vi "TTA_MATLAB_RxACPRTest.vi"(1 "Instrument Cluster In":T2, 11 "error in":errorcluster) -> (4 "ACPR\nResults":T1, 12 "Instrument Cluster Out":T2, 15 "error out":errorcluster)   [LabVIEW 2016]
uses:
  TTA_Globals/TTA_Global_Complete_Settings.vi
  TTA_Controls/TTA_Control_Complete_Settings_Cluster.ctl
  TTA_Controls/TTA_Control_Instrument_Cluster.ctl
panel:
  out "Test Status":string
  in  "Complete Settings Cluster":T3
  out "RFICs":i32[](array[numeric])
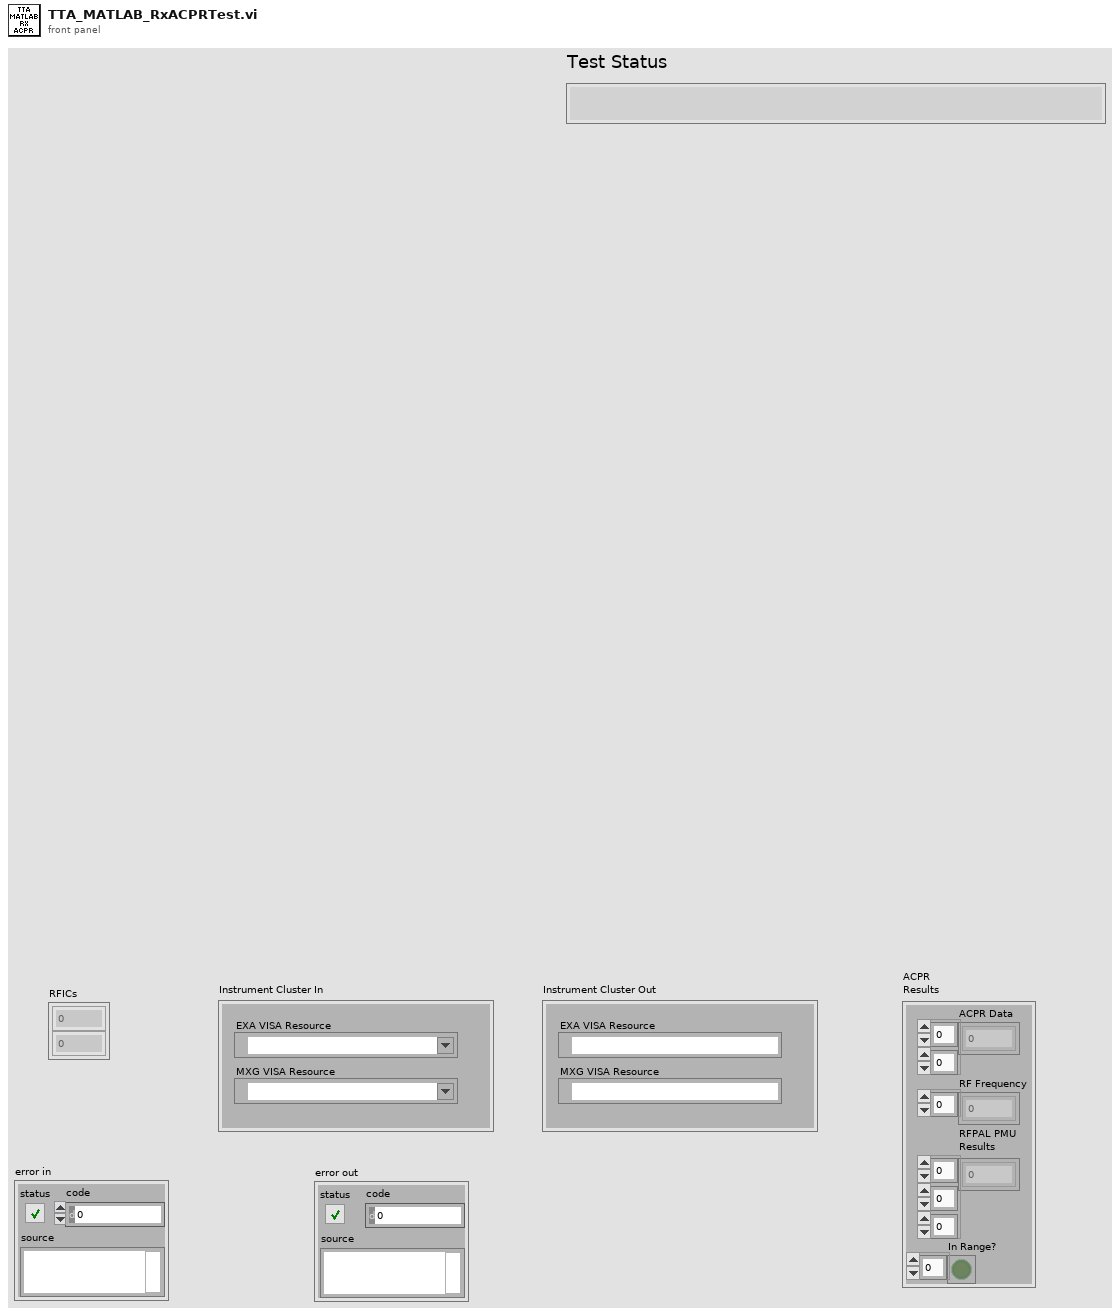
[diagram p1: front panel]
types:
  T1 = cluster{"ACPR Data":dbl[][], "RF Frequency":dbl[], "RFPAL PMU\nResults":dbl[][][], "In Range?":bool[]}
  T2 = typedef "TTA_Control_Instrument_Cluster.ctl" = cluster{"EXA VISA Resource":refnum<visa-resource-name>, "MXG VISA Resource":refnum<visa-resource-name>}
  T3 = typedef "TTA_Control_Complete_Settings_Cluster.ctl" = cluster{"Brief Cluster":cluster{"STM Firmware File":string, "STM Firmware Address":string, "Required SW Version":string, "Template Used":string}, "Instrument Setting Cluster":cluster{"BDSFreq":dbl, "BDS Amp":dbl, "TxRFCal_Freq":dbl, "TxRFCal_Amp":dbl, "RxRFCal_Freq":dbl, "RxRFCal_Freq":dbl, "TxIF_Freq":dbl, "TxIF_Amp":dbl, "Tx_Output_Power_Signal_Freq":dbl, "Tx_ACPR_Signal_Freq":dbl, "Rx_RF_Freq":dbl, "Rx_RF_Amp":dbl, "Rx_Output_Power_Signal_Freq":dbl, "Rx_Output_Power_Sense_Freq":dbl}, "PAL Calibration\nInputs Cluster":cluster{"Amplitude Range\nMax(dBm)":dbl, "Amplitude Range\nMin(dBm)":dbl, "Amplitude Least\nCriteria (dBm)":dbl, "Frequency 1":dbl, "Frequency 2":dbl, "Frequency 3":dbl, "CAL Amplitude\nDecrement (dB)":dbl, "CAL Amplitude\nIncrement(dB)":dbl, "DownloadFile":string}, "TxOffset Cal Cluster":cluster{"Tx1 Offset (dB)":dbl, "Tx2 Offset (dB)":dbl, "Tx3 Offset (dB)":dbl, "Tx4 Offset (dB)":dbl, "Total RF Tx Loss (dB)":dbl}, "RxOffset Cal Cluster":cluster{"Rx1 Offset (dB)":dbl, "Rx2 Offset (dB)":dbl, "Rx3 Offset (dB)":dbl, "Rx4 Offset (dB)":dbl, "Total RF Rx Loss (dB)":dbl}, "TX Output Power Settings Cluster":cluster{"Frequency Sweep (MHz)":dbl[], "Sig Gen \nPower (dBm)":dbl, "Span (kHz)":dbl, "RBW (Hz)":dbl, "Ref Level (dBm)":dbl, "Low Power \nLimit":dbl, "High Power \nLimit":dbl, "DigAtt Max":dbl, "DigAtt Min":dbl}, "Tx ACPR Settings Cluster":cluster{"ACPR Filename":string, "Sampling Rate":dbl, "Power (dBm)":dbl, "IF Frequency Sweep (MHz)":dbl[], "State Name":string, "Mechanical\nAttenuation":dbl, "RefLevel Offset":dbl, "Amplitude Range\nMax (dBm)":dbl, "Amplitude Range\nMin (dBm)":dbl, "Cal Amp \nIncrement (dB)":dbl, "Cal Amp\nDecrement (dB)":dbl}, "Power Cal Cluster":cluster{"Power List (dBm)":dbl[], "Frequency (MHz)":dbl[], "Cal Decrement (dB)":dbl, "Cal Increment (dB)":dbl}, "Rx Received Power Settings Cluster":cluster{"Frequency Sweep (MHz)":dbl[], "Power (dBm)":dbl, "Span (kHz)":dbl, "RBW (Hz)":dbl, "Ref Level":dbl, "Low Power \nLimit (dBm)":dbl, "High Power\nLimit (dBm)":dbl}, "Tx Output Power Criteria Cluster":cluster{"CH1-TX1 \nMin":dbl, "CH1-TX1\nMax":dbl, "CH1-TXx3\nMin ":dbl, "CH1-TXx3\nMax":dbl, "CH2-TX1\nMin":dbl, "CH2-TX1\nMax":dbl, "CH2-TXx3\nMin":dbl, "CH2-TXx3\nMax":dbl}, "Tx ACPR Criteria Cluster":cluster{"Min Inband":dbl, "Max Close Outband":dbl, "Max Far Outband":dbl}, "Rx Output Power Criteria Cluster":cluster{"CH1-RX1 \nMin":dbl, "CH1-RX1 \nMax":dbl, "CH1-RXx3 \nMin":dbl, "CH1-RXx3\nMax":dbl, "CH2-RX1\nMin":dbl, "CH2-RX1\nMax":dbl, "CH2-RXx3\nMin":dbl, "CH2-RXx3\nMax":dbl}}
  T4 = cluster{"Amplitude Range\nMax(dBm)":dbl, "Amplitude Range\nMin(dBm)":dbl, "Amplitude Least\nCriteria (dBm)":dbl, "Frequency 1":dbl, "Frequency 2":dbl, "Frequency 3":dbl, "CAL Amplitude\nDecrement (dB)":dbl, "CAL Amplitude\nIncrement(dB)":dbl, "DownloadFile":string}
  T5 = cluster{"ACPR Filename":string, "Sampling Rate":dbl, "Power (dBm)":dbl, "IF Frequency Sweep (MHz)":dbl[], "State Name":string, "Mechanical\nAttenuation":dbl, "RefLevel Offset":dbl, "Amplitude Range\nMax (dBm)":dbl, "Amplitude Range\nMin (dBm)":dbl, "Cal Amp \nIncrement (dB)":dbl, "Cal Amp\nDecrement (dB)":dbl}
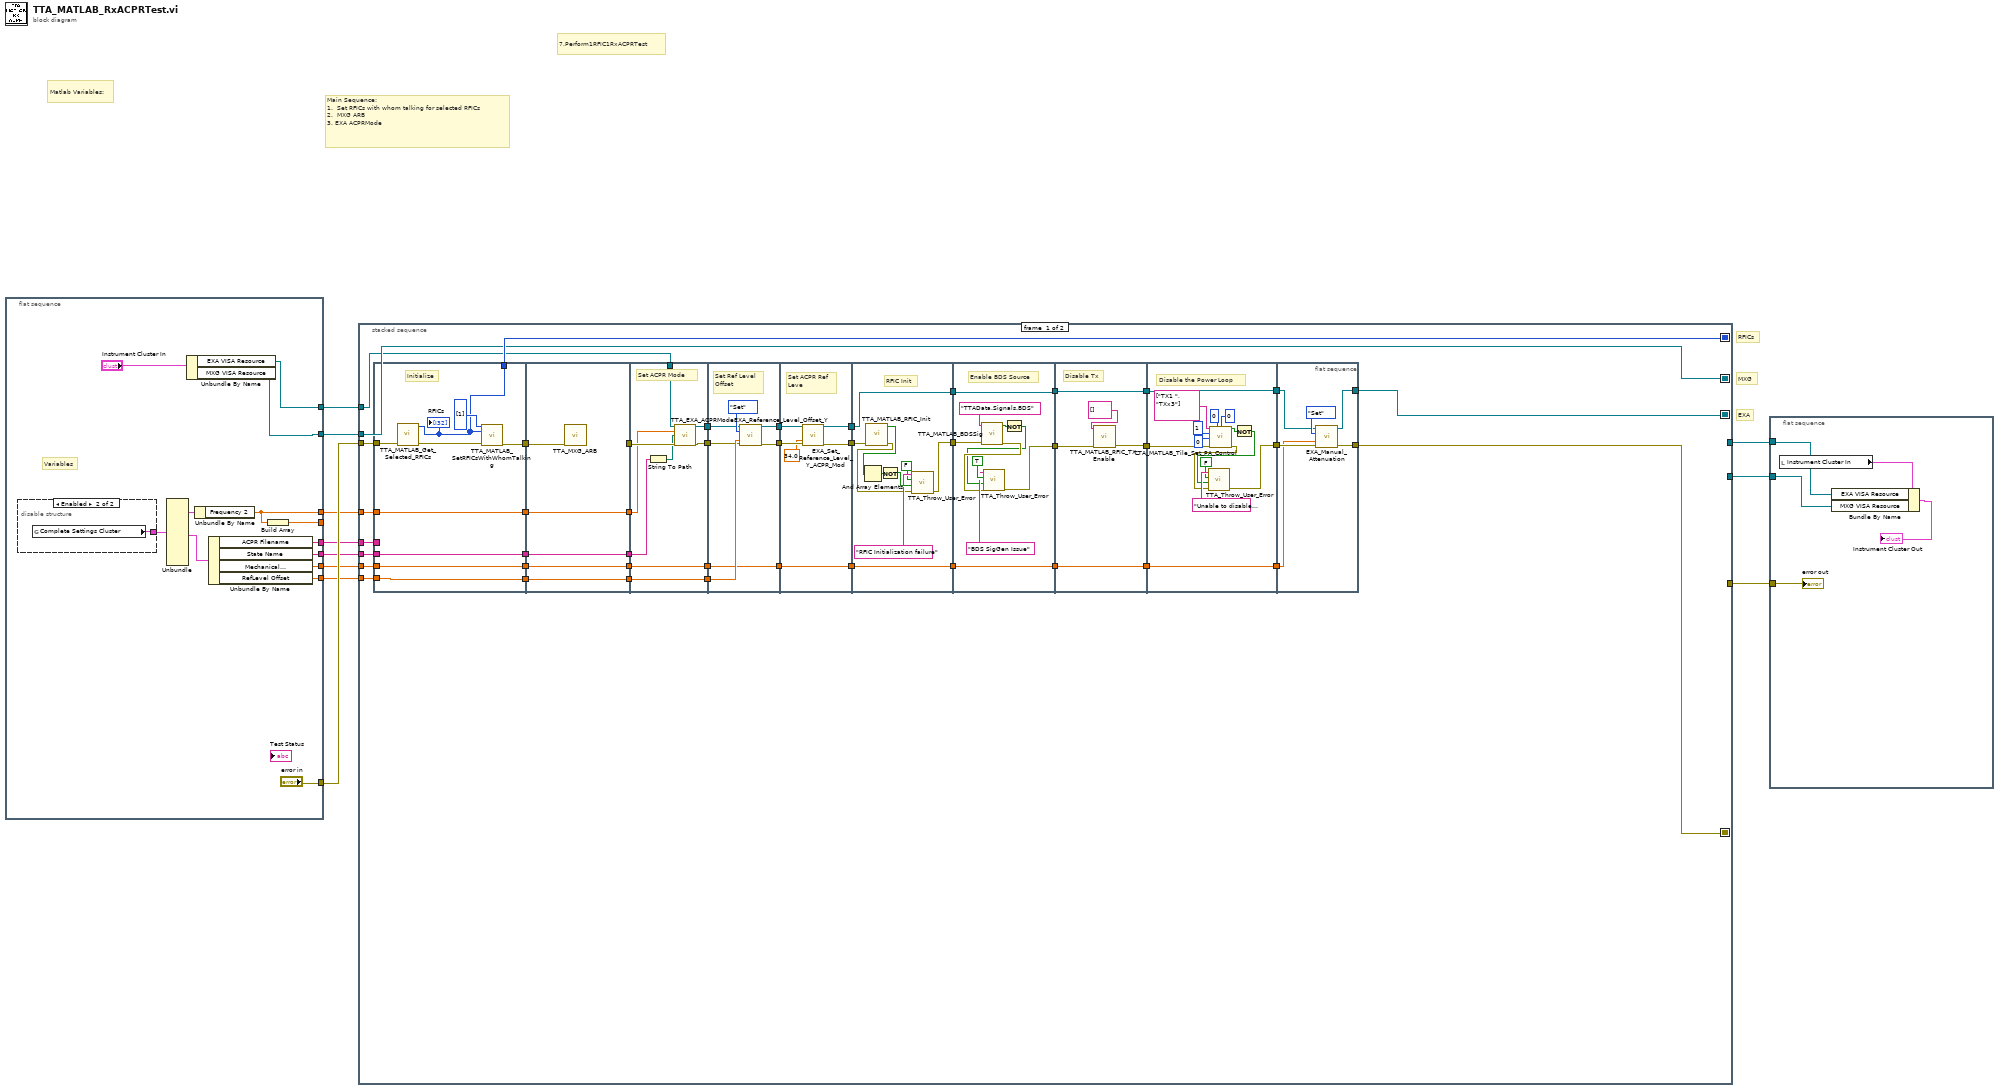
[diagram p0: block diagram]
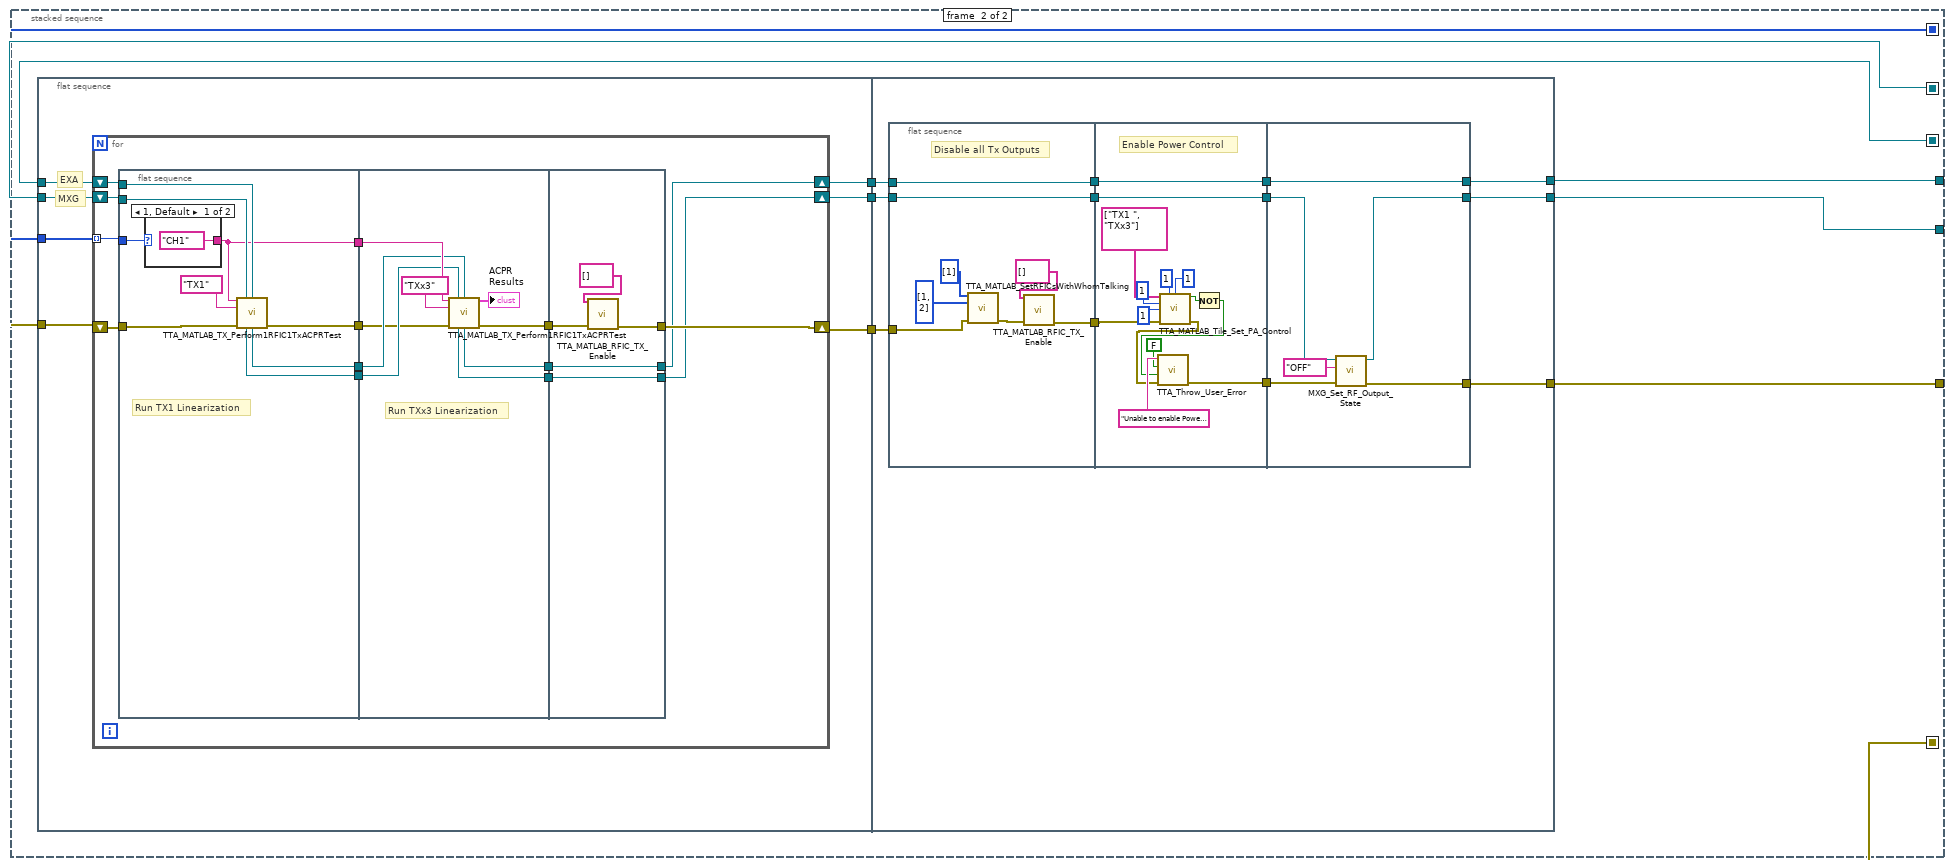
[diagram p2: hidden frame]
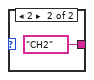
[diagram p3: hidden frame]
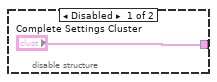
[diagram p4: hidden frame]
diagram:
  # "RFICs"
  # "EXA"
  # "MXG"
  # "Matlab Variables:"
  # "Main Sequence:\n1.  Set RFICs with whom talking for selected RFICs\n2.  MXG ARB\n3. EXA ACPRMode"
  # "7.Perform1RFIC1RxACPRTest"
  n1 = flat-sequence {
    tunnel: ["error in"] -> w11
    tunnel: [w19] -> w10
    tunnel: [w18] -> w9
    tunnel: [w22] -> _
    tunnel: [w17] -> w5
    tunnel: [w15] -> w4
    tunnel: [w14] -> w3
    tunnel: [w13] -> w2
    tunnel: [w12] -> w1
    frame #0 {
      # "Variables"
      n2 = disable-structure shown="Enabled" {
        disable-tunnel: ["Complete Settings Cluster" w26] -> w24
        frame Disabled {
        }
        frame Enabled {
          n3 = global read "TTA_Global_Complete_Settings.vi" "Complete Settings Cluster"() -> (w26:T3)
        }
      }
      n4 = Unbundle(w24) -> ("PAL Calibration\nInputs Cluster"=w21:T4, "Tx ACPR Settings Cluster"=w16:T5)  [unwired: 10 out]
      n5 = Unbundle By Name("Instrument Cluster In") -> ("EXA VISA Resource"=w19:refnum<visa-resource-name>, "MXG VISA Resource"=w18:refnum<visa-resource-name>)
      n6 = Unbundle By Name(w21) -> ("Frequency 2"=w17:dbl)
      n7 = Unbundle By Name(w16) -> ("ACPR Filename"=w12:string, "State Name"=w15:string, "Mechanical\nAttenuation"=w14:dbl, "RefLevel Offset"=w13:dbl)
      n8 = Build Array(w17) -> (w22:dbl[])
    }
  }
  n9 = stacked-sequence {
    seq-local: [w68 _] -> [_ w160]
    seq-local: [w50 _] -> [_ w158]
    seq-local: [w62 _] -> [_ w159]
    seq-local: [w66 _] -> [_ w157]
    tunnel: w11 -> [w69 _]
    tunnel: w10 -> [w64 _]
    tunnel: w9 -> [w66 _]
    tunnel: [_ w154] -> w8
    tunnel: [_ w153] -> w7
    tunnel: [_ w152] -> w6
    tunnel: w5 -> [w65 _]
    tunnel: w4 -> [w61 _]
    tunnel: w3 -> [w60 _]
    tunnel: w2 -> [w59 _]
    tunnel: w1 -> [w27 _]
    frame #0 {
      n10 = flat-sequence {
        tunnel: w69 -> [w76]
        tunnel: [w75] -> w68
        tunnel: [w74] -> w37
        tunnel: w65 -> [w73]
        tunnel: [w73] -> w35
        tunnel: w61 -> [w72]
        tunnel: [w72] -> w33
        tunnel: w60 -> [w71]
        tunnel: [w71] -> w31
        tunnel: w59 -> [w70]
        tunnel: [w70] -> w29
        tunnel: w27 -> [_]
        tunnel: w37 -> [w79]
        tunnel: [_] -> w36
        tunnel: w35 -> [w83]
        tunnel: [w83] -> w34
        tunnel: w33 -> [w82]
        tunnel: [w82] -> w32
        tunnel: w31 -> [w81]
        tunnel: [w81] -> w30
        tunnel: w29 -> [w80]
        tunnel: [w80] -> w28
        tunnel: w36 -> [w92]
        tunnel: w34 -> [w90]
        tunnel: w64 -> [w91]
        tunnel: w32 -> [w89]
        tunnel: w30 -> [w84]
        tunnel: [w87] -> w41
        tunnel: w28 -> [w87]
        tunnel: [w86] -> w40
        tunnel: [w85] -> w39
        tunnel: [w84] -> w38
        tunnel: [w96] -> w58
        tunnel: [w97] -> w56
        tunnel: w41 -> [w99]
        tunnel: [w93] -> w47
        tunnel: w40 -> [w95]
        tunnel: w39 -> [w94]
        tunnel: w38 -> [w93]
        tunnel: w58 -> [w105]
        tunnel: [w102] -> w57
        tunnel: w56 -> [w104]
        tunnel: [w103] -> w55
        tunnel: w47 -> [w100]
        tunnel: [w100] -> w42
        tunnel: w57 -> [w110]
        tunnel: [w108] -> w67
        tunnel: w55 -> [w107]
        tunnel: [w107] -> w63
        tunnel: [w106] -> w43
        tunnel: w42 -> [w106]
        tunnel: w67 -> [w121]
        tunnel: w63 -> [w118]
        tunnel: [w118] -> w54
        tunnel: [w117] -> w52
        tunnel: [w116] -> w44
        tunnel: w43 -> [w116]
        tunnel: w54 -> [w130]
        tunnel: [w130] -> w53
        tunnel: w52 -> [w128]
        tunnel: [w127] -> w51
        tunnel: [w126] -> w45
        tunnel: w44 -> [w126]
        tunnel: w53 -> [w135]
        tunnel: w51 -> [w134]
        tunnel: [w135] -> w49
        tunnel: [w132] -> w48
        tunnel: [w131] -> w46
        tunnel: w45 -> [w131]
        tunnel: [w148] -> w50
        tunnel: [w146] -> w62
        tunnel: w49 -> [w147]
        tunnel: w48 -> [w149]
        tunnel: w46 -> [w145]
        frame #0 {
          # "Initialize"
          n11 = call "TTA_MATLAB_Get_Selected_RFICs.vi"("error in"=w76) -> ("RFICs"=w75:i32[], "error out"=w77:errorcluster)  [unwired: 13 in]
          "RFICs" <- w75
          n12 = call "TTA_MATLAB_SetRFICsWithWhomTalking.vi"("Panel Array"=i32[] [1], "RFIC Array"=w75, "error in"=w77) -> ("error out"=w74:errorcluster)  [unwired: 12 in]
        }
        frame #1 {
          n13 = call "TTA_MXG_ARB.vi"("error in"=w79) -> ()  [unwired: 13 in, 2 out]
        }
        frame #2 {
          # "Set ACPR Mode"
          n14 = String To Path(string=w89) -> (path=w88:path)
          n15 = call "TTA_EXA_ACPRMode.vi"("VISA resource In"=w91, "Frequency (MHz)"=w90, "State File"=w88, "error in"=w92) -> ("VISA resource Out"=w85:refnum<visa-resource-name>, "error out"=w86:errorcluster)  [unwired: 10 in]
        }
        frame #3 {
          # "Set Ref Level \nOffset"
          n16 = call "EXA_Reference_Level_Offset_Y.vi"("VISA resource name"=w94, "Mode"=enum16{"Set", "Get"}."Set", "Reference Level \nOffset (dBm)"=w99, "error in"=w95) -> ("VISA resource name"=w97:refnum<visa-resource-name>, "error out"=w96:errorcluster)  [unwired: 9 in, 1 out]
        }
        frame #4 {
          # "Set ACPR Ref\nLeve"
          n17 = call "EXA_Set_Reference_Level_Y_ACPR_Mod.vi"("VISA resource name"=w104, "Reference Level \nOffset (dBm)"=34.0 ("Reference Level \nOffset (dBm)"), "error in"=w105) -> ("VISA resource name"=w103:refnum<visa-resource-name>, "error out"=w102:errorcluster)  [unwired: 11 in]
        }
        frame #5 {
          # "RFIC Init"
          n18 = call "TTA_MATLAB_RFIC_Init.vi"("error in"=w110) -> ("SuccessComm"=w115:bool[], "error out"=w109:errorcluster)  [unwired: 13 in]
          n19 = And Array Elements(Boolean array=w115) -> (logical AND=w114:bool)
          n20 = Not(x=w114) -> (.not. x?=w113:bool)
          n21 = call "TTA_Throw_User_Error.vi"("error in"=w109, "Error?"=w113, "Stop Execution on Fail"=FALSE, "Error Message"="RFIC Initialization failure") -> ("error out"=w108:errorcluster)  [unwired: 7 in]
        }
        frame #6 {
          # "Enable BDS Source"
          n22 = call "TTA_MATLAB_BDSSig.vi"("Signal Settings"="TTAData.Signals.BDS", "error in"=w121) -> ("Success"=w122:bool, "error out"=w120:errorcluster)  [unwired: 12 in]
          n23 = Not(x=w122) -> (.not. x?=w119:bool)
          n24 = call "TTA_Throw_User_Error.vi"("error in"=w120, "Error?"=w119, "Stop Execution on Fail"=TRUE, "Error Message"="BDS SigGen Issue") -> ("error out"=w117:errorcluster)  [unwired: 7 in]
        }
        frame #7 {
          # "Disable Tx"
          n25 = call "TTA_MATLAB_RFIC_TX_Enable.vi"("Channels"=string[] [], "error in"=w128) -> ("error out"=w127:errorcluster)  [unwired: 12 in, 1 out]
        }
        frame #8 {
          # "Disable the Power Loop"
          n26 = call "TTA_MATLAB_Tile_Set_PA_Control.vi"("Channels"=string[] ["TX1 ", "TXx3"], "OutPower"=0, "InPower"=0, "Temp"=1, "Current"=0, "error in"=w134) -> ("Success"=w138:bool, "error out"=w136:errorcluster)  [unwired: 6 in, 2 out]
          n27 = Not(x=w138) -> (.not. x?=w137:bool)
          n28 = call "TTA_Throw_User_Error.vi"("error in"=w136, "Error?"=w137, "Stop Execution on Fail"=FALSE, "Error Message"="Unable to disable Power Loop") -> ("error out"=w132:errorcluster)  [unwired: 7 in]
        }
        frame #9 {
          n29 = call "EXA_Manual_Attenuation.vi"("VISA resource name"=w147, "Mode"=enum16{"Set", "Get"}."Set", "Attenuation (dB)"=w145, "error in"=w149) -> ("VISA resource name"=w146:refnum<visa-resource-name>, "error out"=w148:errorcluster)  [unwired: 9 in, 1 out]
        }
      }
    }
    frame #1 {
      n30 = flat-sequence {
        tunnel: w160 -> [w165]
        tunnel: w159 -> [w167]
        tunnel: w157 -> [w166]
        tunnel: w158 -> [w164]
        tunnel: [w162] -> w156
        tunnel: [w161] -> w155
        tunnel: [w163] -> w151
        tunnel: w156 -> [w217]
        tunnel: w155 -> [w216]
        tunnel: [w209] -> w154
        tunnel: [w208] -> w153
        tunnel: [w207] -> w152
        tunnel: w151 -> [w218]
        frame #0 {
          # "EXA"
          # "MXG"
          n31 = for {
            tunnel: w165 -> [w176] mode=indexing
            shift-right: [w170] -> w163
            shift-left: w164 -> [w171]
            shift-right: [w169] -> w162
            shift-left: w167 -> [w178]
            shift-right: [w168] -> w161
            shift-left: w166 -> [w177]
            n32 = flat-sequence {
              tunnel: w176 -> [w190]
              tunnel: w178 -> [w188]
              tunnel: w177 -> [w187]
              tunnel: w171 -> [w186]
              tunnel: [w185] -> w175
              tunnel: [w184] -> w174
              tunnel: [w183] -> w173
              tunnel: [w182] -> w172
              tunnel: w175 -> [w200]
              tunnel: w174 -> [w198]
              tunnel: w173 -> [w197]
              tunnel: [w199] -> w181
              tunnel: [w196] -> w180
              tunnel: [w195] -> w179
              tunnel: w172 -> [w194]
              tunnel: [w205] -> w169
              tunnel: [w206] -> w168
              tunnel: w181 -> [w203]
              tunnel: w180 -> [w206]
              tunnel: w179 -> [w205]
              tunnel: [w202] -> w170
              frame #0 {
                # "Run TX1 Linearization"
                n33 = case shown="1, Default" w190 {
                  tunnel: ["CH1" ("Channel") "CH2" ("Channel")] -> w185
                  frame 1, Default {
                  }
                  frame 2 {
                  }
                }
                n34 = call "TTA_MATLAB_TX_Perform1RFIC1TxACPRTest.vi"("Channel"=w185, "MXG VISA Resource In"=w187, "EXA VISA Resource"=w188, "Tx"="TX1", "error in"=w186) -> ("MXG VISA Resource Out"=w184:refnum<visa-resource-name>, "EXA VISA Resource Out"=w183:refnum<visa-resource-name>, "error out"=w182:errorcluster)  [unwired: 7 in, 1 out]
              }
              frame #1 {
                # "Run TXx3 Linearization"
                n35 = call "TTA_MATLAB_TX_Perform1RFIC1TxACPRTest.vi"("Channel"=w200, "MXG VISA Resource In"=w198, "EXA VISA Resource"=w197, "Tx"="TXx3", "error in"=w194) -> ("ACPR\nResults"=→"ACPR\nResults":T1, "MXG VISA Resource Out"=w196:refnum<visa-resource-name>, "EXA VISA Resource Out"=w195:refnum<visa-resource-name>, "error out"=w199:errorcluster)  [unwired: 7 in]
              }
              frame #2 {
                n36 = call "TTA_MATLAB_RFIC_TX_Enable.vi"("Channels"=string[] [], "error in"=w203) -> ("error out"=w202:errorcluster)  [unwired: 12 in, 1 out]
              }
            }
          }
        }
        frame #1 {
          n37 = flat-sequence {
            tunnel: w218 -> [w224]
            tunnel: w217 -> [w220]
            tunnel: w216 -> [w219]
            tunnel: [w221] -> w215
            tunnel: [w220] -> w214
            tunnel: [w219] -> w213
            tunnel: w215 -> [w229]
            tunnel: w214 -> [w240]
            tunnel: w213 -> [w239]
            tunnel: [w240] -> w212
            tunnel: [w239] -> w211
            tunnel: [w227] -> w210
            tunnel: [w243] -> w208
            tunnel: [w246] -> w207
            tunnel: w212 -> [w246]
            tunnel: w211 -> [w244]
            tunnel: w210 -> [w245]
            tunnel: [w241] -> w209
            frame #0 {
              # "Disable all Tx Outputs"
              n38 = call "TTA_MATLAB_SetRFICsWithWhomTalking.vi"("Panel Array"=i32[] [1], "RFIC Array"=i32[] [1, 2], "error in"=w224) -> ("error out"=w222:errorcluster)  [unwired: 12 in]
              n39 = call "TTA_MATLAB_RFIC_TX_Enable.vi"("Channels"=string[] [], "error in"=w222) -> ("error out"=w221:errorcluster)  [unwired: 12 in, 1 out]
            }
            frame #1 {
              # "Enable Power Control"
              n40 = call "TTA_MATLAB_Tile_Set_PA_Control.vi"("Channels"=string[] ["TX1 ", "TXx3"], "OutPower"=1, "InPower"=1, "Temp"=1, "Current"=1, "error in"=w229) -> ("Success"=w232:bool, "error out"=w230:errorcluster)  [unwired: 6 in, 2 out]
              n41 = Not(x=w232) -> (.not. x?=w231:bool)
              n42 = call "TTA_Throw_User_Error.vi"("error in"=w230, "Error?"=w231, "Stop Execution on Fail"=FALSE, "Error Message"="Unable to enable Power Loop") -> ("error out"=w227:errorcluster)  [unwired: 7 in]
            }
            frame #2 {
              n43 = call "MXG_Set_RF_Output_State.vi"("error in"=w245, "RF Output State"="OFF", "VISA resource name"=w244) -> ("error out"=w241:errorcluster, "VISA resource name"=w243:refnum<visa-resource-name>)  [unwired: 7 in]
            }
          }
        }
      }
    }
  }
  n44 = flat-sequence {
    tunnel: w8 -> [w251]
    tunnel: w7 -> [w248]
    tunnel: w6 -> [w249]
    frame #0 {
      n45 = local read "Instrument Cluster In"() -> (w247:T2)
      n46 = Bundle By Name(cluster=w247, "EXA VISA Resource"=w249, "MXG VISA Resource"=w248) -> (→"Instrument Cluster Out":T2)
      "error out" <- w251
    }
  }
